vi "Set Current.vi"(0 "reference in":refnum<class "Simulated-PowerModule.lvclass">, 5 "current (A)":dbl, 11 "Error In":errorcluster) -> (4 "reference out":refnum<class "Simulated-PowerModule.lvclass">, 15 "Error Out":errorcluster)   [LabVIEW 2023, in "Simulated-PowerModule.lvlib" / "Simulated-PowerModule.lvclass"]
uses:
  Simulated-PowerModule.lvclass
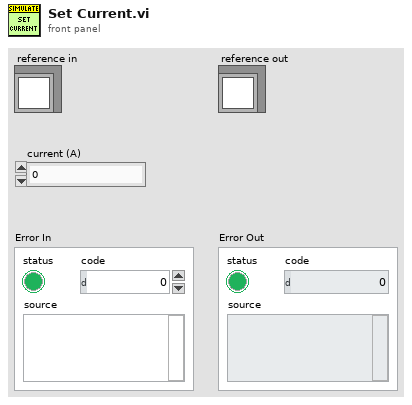
[diagram p1: front panel]
types:
  T1 = typedef "Simulated-PowerModule.lvlib/Simulated-PowerModule.lvclass/ObjectAttributes.ctl" = cluster{"JSON Config Path":path, "Configuration":T2, "connected":bool, "reserved":bool, "energized":bool, "output enabled":bool, "setpoint":cluster{"voltage":sgl, "current":sgl, "resistance":sgl}, "last timestamp":i64, "mode":T4, "range":T3, "measurement array":T5[], "profile":dbl[][], "step dt":i64}
  T2 = typedef "Simulated-PowerModule.lvlib/Simulated-PowerModule.lvclass/Configuration.ctl" = cluster{"range":T3}
  T3 = typedef "PowerModuleInterface.lvlibp/PowerModuleInterface.lvclass/Range.ctl" = cluster{"Current Max (A)":dbl, "Current Min (A)":dbl, "Voltage Max (V)":dbl, "Voltage Min (V)":dbl}
  T4 = typedef "Simulated-PowerModule.lvlib/Simulated-PowerModule.lvclass/Mode.ctl" = u16
  T5 = typedef "PowerModuleInterface.lvlibp/PowerModuleInterface.lvclass/Measurements.ctl" = cluster{"measured voltage (V)":dbl, "measured current (A)":dbl, "setpoint voltage (V)":dbl, "setpoint current (A)":dbl, "timestamp":dbl}
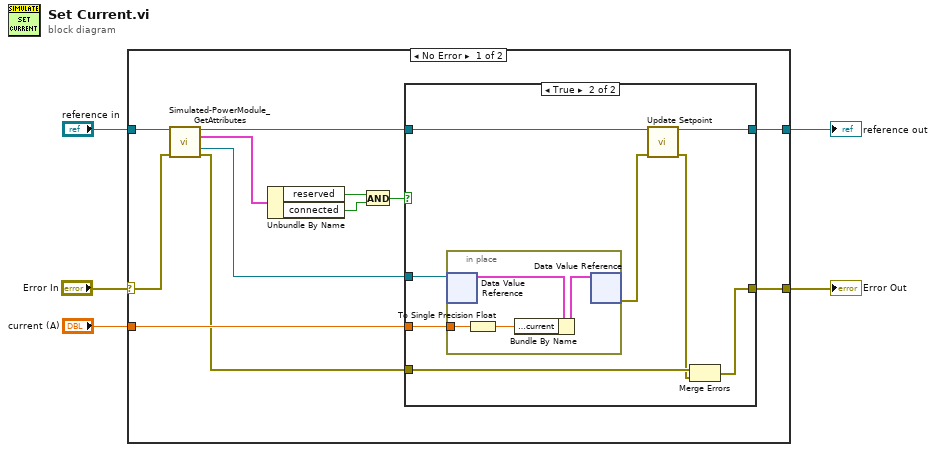
[diagram p0: block diagram]
diagram:
  n1 = case shown="No Error" "Error In" {
    selector: "Error In" -> [w16 w32]
    tunnel: "reference in" -> [w17 w33]
    tunnel: [w13 w33] -> w3
    tunnel: [w12 w32] -> w2
    tunnel: "current (A)" -> [w11 _]
    frame No Error {
      n2 = call "Simulated-PowerModule_GetAttributes.vi"("reference in"=w17, "Error In"=w16) -> ("reference out"=w14:refnum<class "Simulated-PowerModule.lvclass">, "Data"=w10:T1, "DataRef"=w15:refnum<data-value>, "Error Out"=w9:errorcluster)  [unwired: 10 in]
      n3 = Unbundle By Name(w10) -> ("reserved"=w8:bool, "connected"=w7:bool)
      n4 = And(x=w8, y=w7) -> (x .and. y?=w6:bool)
      n5 = case shown="True" w6 {
        tunnel: w15 -> [_ w27]
        tunnel: w14 -> [w19 w26]
        tunnel: [w19 w25] -> w13
        tunnel: [w18 w20] -> w12
        tunnel: w11 -> [_ w24]
        tunnel: w9 -> [w18 w23]
        frame False {
        }
        frame True {
          n6 = in-place {
            in-place-border: w24 -> [w29]
            n7 = in-place-dvr #1(w27) -> (w31:T1)  [unwired: 1 out]
            n8 = To Single Precision Float(number=w29) -> (single precision float=w28:sgl)
            n9 = Bundle By Name(cluster=w31, "setpoint.current"=w28) -> (w30:T1)
            n10 = in-place-dvr #1(w30) -> (w22:errorcluster)  [unwired: 1 out]
          }
          n11 = call "Update Setpoint.vi"("reference in"=w26, "Error In"=w22) -> ("reference out"=w25:refnum<class "Simulated-PowerModule.lvclass">, "Error Out"=w21:errorcluster)  [unwired: 12 in]
          n12 = Merge Errors(w23, w21) -> (w20:errorcluster)
        }
      }
    }
    frame Error {
    }
  }
  "Error Out" <- w2
  "reference out" <- w3
